vi "testSendTelToClientAndCmdToServer.vi"(8 "error in (no error)":errorcluster) -> (0 "error out":errorcluster)   [LabVIEW 2018]
doc: "This VI sends commands from TCP client and receives the Ack from TCP server. Besides, TCP server sends telemetry to TCP client."
uses:
  <vilib>/addons/_JKI Toolkits/Caraya/classes/Assert/Assert Equal Value_Variant.vi
  src/TcpServer/TcpServer.lvclass
  <vilib>/addons/_JKI Toolkits/Caraya/classes/Test/Test.lvclass
  <vilib>/addons/_JKI Toolkits/Caraya/classes/Assert/Assert.lvclass
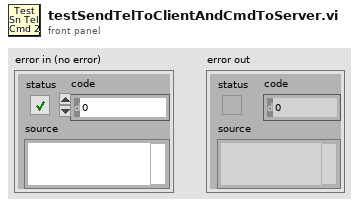
[diagram p1: front panel]
types:
  T1 = cluster{"CmdRead":refnum<user-event>, "EvtRead":refnum<user-event>, "GenRead":refnum<user-event>}
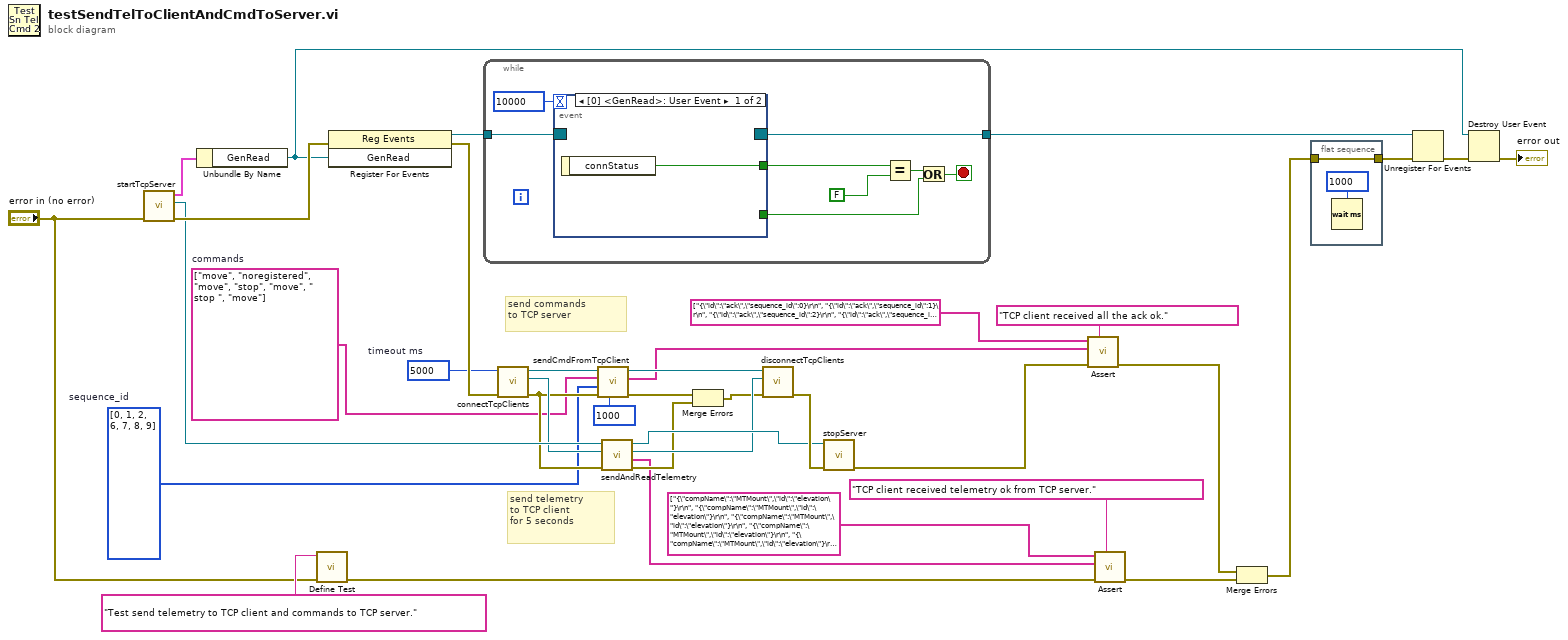
[diagram p0: block diagram]
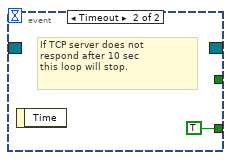
[diagram p2: hidden frame]
diagram:
  w3 = i32[] [0, 1, 2, 6, 7, 8, 9]  # sequence_id
  w4 = string[] ["move", "noregistered", "move", "stop", "move", " stop ", "move"]  # commands
  w6 = 5000  # timeout ms
  # "send commands\nto TCP server"
  # "send telemetry\nto TCP client\nfor 5 seconds"
  n1 = call "startTcpServer.vi"("error in (no error)"="error in (no error)") -> ("error out"=w31:errorcluster, "TcpServer out"=w17:refnum<class "TcpServer.lvclass">, "UserEvents"=w32:T1)  [unwired: 8 in]
  n2 = Unbundle By Name(w32) -> ("GenRead"=w1:refnum<user-event>)
  n3 = call <vilib>:"Define Test.vi"("error in (no error)"="error in (no error)", "Label (VI Title)"="Test send telemetry to TCP client and commands to TCP server.") -> ("error out"=w29:errorcluster)  [unwired: 9 in]
  n4 = register-events(error in=w31, w1) -> (reference out=w37:refnum<event-registration>, error out=w7:errorcluster)  [unwired: 1 in]
  n5 = while {
    tunnel: w37 -> [w45]
    tunnel: [w44] -> w36
    stop <- w42 stop-if-true
    n6 = event shown="[0] <GenRead>: User Event" {
      selector: w45 -> [_ _]
      dyn-events: [_ _] -> w44
      timeout: 10000 -> [_ _]
      tunnel: [w46 _] -> w43
      tunnel: [_ TRUE] -> w39
      event User Event {
        n7 = event-data() -> ("connStatus"=w46:bool)  [unwired: 1 in]
      }
      event Timeout {
        # "If TCP server does not\nrespond after 10 sec\nthis loop will stop."
        n8 = event-data() -> ()  [unwired: 1 in, 1 out]
      }
    }
    n9 = Equal?(x=w43, y=FALSE) -> (x = y?=w40:bool)
    n10 = Or(x=w40, y=w39) -> (x .or. y?=w42:bool)
  }
  n11 = call "connectTcpClients.vi"("error in (no error)"=w7, "timeout ms"=w6) -> ("error out"=w8:errorcluster, "tel connection ID out"=w15:refnum<k5>, "cmd connection ID out"=w25:refnum<k5>)  [unwired: 7 in]
  n12 = call "sendCmdFromTcpClient.vi"("timeout ms (1000)"=1000, "error in (no error)"=w8, "sequence_id"=w3, "commands"=w4, "connectionID"=w25) -> ("error out"=w21:errorcluster, "ack received"=w18:string[], "connectionID"=w22:refnum<k5>)  [unwired: 4 in]
  n13 = call "sendAndReadTelemetry.vi"("error in (no error)"=w8, "tel connection in"=w15, "TcpServer out"=w17) -> ("error out"=w13:errorcluster, "telemetry received"=w12:string[], "tel connection out"=w14:refnum<k5>, "tcpServer out"=w16:refnum<class "TcpServer.lvclass">)  [unwired: 5 in]
  n14 = Merge Errors(w21, w13) -> (w10:errorcluster)
  n15 = call "disconnectTcpClients.vi"("error in (no error)"=w10, "tel connection ID in"=w14, "cmd connection ID in"=w22) -> ("error out"=w20:errorcluster)  [unwired: 8 in]
  n16 = call "stopServer.vi"("error in (no error)"=w20, "tcpServer in"=w16) -> ("error out"=w19:errorcluster)  [unwired: 8 in, 1 out]
  n17 = call-poly <vilib>:"Assert.vi"("Label"="TCP client received all the ack ok.", "error in (no error)"=w19, "Y"=w18, "X"=string[] ["{\"id\":\"ack\",\"sequence_id\":0}\r\n", "{\"id\":\"ack\",\"sequence_id\":1}\r\n", "{\"id\":\"ack\",\"sequence_id\":2}\r\n", "{\"id\":\"ack\",\"sequence_id\":6}\r\n", "{\"id\":\"noack\",\"sequence_id\":3}\r\n", "{\"id\":\"noack\",\"sequence_id\":4}\r\n", "{\"id\":\"noack\",\"sequence_id\":5}\r\n", "{\"id\":\"ack\",\"sequence_id\":7}\r\n", "{\"id\":\"ack\",\"sequence_id\":8}\r\n", "{\"id\":\"ack\",\"sequence_id\":9}\r\n"] ("ack received 2")) -> ("error out"=w23:errorcluster)  [unwired: 7 in]
  n18 = call-poly <vilib>:"Assert.vi"("Label"="TCP client received telemetry ok from TCP server.", "error in (no error)"=w29, "Y"=w12, "X"=string[] ["{\"compName\":\"MTMount\",\"id\":\"elevation\"}\r\n", "{\"compName\":\"MTMount\",\"id\":\"elevation\"}\r\n", "{\"compName\":\"MTMount\",\"id\":\"elevation\"}\r\n", "{\"compName\":\"MTMount\",\"id\":\"elevation\"}\r\n", "{\"compName\":\"MTMount\",\"id\":\"elevation\"}\r\n", "{\"compName\":\"MTMount\",\"id\":\"elevation\"}\r\n", "{\"compName\":\"MTMount\",\"id\":\"elevation\"}\r\n", "{\"compName\":\"MTMount\",\"id\":\"elevation\"}\r\n", "{\"compName\":\"MTMount\",\"id\":\"elevation\"}\r\n", "{\"compName\":\"MTMount\",\"id\":\"elevation\"}\r\n", "{\"compName\":\"MTMount\",\"id\":\"elevation\"}\r\n", "{\"compName\":\"MTMount\",\"id\":\"elevation\"}\r\n", "{\"compName\":\"MTMount\",\"id\":\"elevation\"}\r\n", "{\"compName\":\"MTMount\",\"id\":\"elevation\"}\r\n", "{\"compName\":\"MTMount\",\"id\":\"elevation\"}\r\n", "{\"compName\":\"MTMount\",\"id\":\"elevation\"}\r\n", "{\"compName\":\"MTMount\",\"id\":\"elevation\"}\r\n", "{\"compName\":\"MTMount\",\"id\":\"elevation\"}\r\n", "{\"compName\":\"MTMount\",\"id\":\"elevation\"}\r\n", "{\"compName\":\"MTMount\",\"id\":\"elevation\"}\r\n", "{\"compName\":\"MTMount\",\"id\":\"elevation\"}\r\n", "{\"compName\":\"MTMount\",\"id\":\"elevation\"}\r\n", "{\"compName\":\"MTMount\",\"id\":\"elevation\"}\r\n", "{\"compName\":\"MTMount\",\"id\":\"elevation\"}\r\n", "{\"compName\":\"MTMount\",\"id\":\"elevation\"}\r\n", "{\"compName\":\"MTMount\",\"id\":\"elevation\"}\r\n", "{\"compName\":\"MTMount\",\"id\":\"elevation\"}\r\n", "{\"compName\":\"MTMount\",\"id\":\"elevation\"}\r\n", "{\"compName\":\"MTMount\",\"id\":\"elevation\"}\r\n", "{\"compName\":\"MTMount\",\"id\":\"elevation\"}\r\n", "{\"compName\":\"MTMount\",\"id\":\"elevation\"}\r\n", "{\"compName\":\"MTMount\",\"id\":\"elevation\"}\r\n", "{\"compName\":\"MTMount\",\"id\":\"elevation\"}\r\n", "{\"compName\":\"MTMount\",\"id\":\"elevation\"}\r\n", "{\"compName\":\"MTMount\",\"id\":\"elevation\"}\r\n", "{\"compName\":\"MTMount\",\"id\":\"elevation\"}\r\n", "{\"compName\":\"MTMount\",\"id\":\"elevation\"}\r\n", "{\"compName\":\"MTMount\",\"id\":\"elevation\"}\r\n", "{\"compName\":\"MTMount\",\"id\":\"elevation\"}\r\n", "{\"compName\":\"MTMount\",\"id\":\"elevation\"}\r\n", "{\"compName\":\"MTMount\",\"id\":\"elevation\"}\r\n", "{\"compName\":\"MTMount\",\"id\":\"elevation\"}\r\n", "{\"compName\":\"MTMount\",\"id\":\"elevation\"}\r\n", "{\"compName\":\"MTMount\",\"id\":\"elevation\"}\r\n", "{\"compName\":\"MTMount\",\"id\":\"elevation\"}\r\n", "{\"compName\":\"MTMount\",\"id\":\"elevation\"}\r\n", "{\"compName\":\"MTMount\",\"id\":\"elevation\"}\r\n", "{\"compName\":\"MTMount\",\"id\":\"elevation\"}\r\n", "{\"compName\":\"MTMount\",\"id\":\"elevation\"}\r\n", "{\"compName\":\"MTMount\",\"id\":\"elevation\"}\r\n"] ("Array 2")) -> ("error out"=w26:errorcluster)  [unwired: 7 in]
  n19 = Merge Errors(w23, w26) -> (w27:errorcluster)
  n20 = flat-sequence {
    tunnel: w27 -> [w48]
    tunnel: [w48] -> w34
    frame #0 {
      n21 = Wait (ms)(milliseconds to wait=u32 1000) -> ()  [unwired: 1 out]
    }
  }
  n22 = Unregister For Events(event registration refnum=w36, error in=w34) -> (error out=w35:errorcluster)
  n23 = Destroy User Event(user event=w1, error in=w35) -> (error out=→"error out":errorcluster)
